vi "getAvailableDevices.vi"(8 "error in (no error)":errorcluster, 11 "IDevice in":refnum<class "IDevice.lvclass">) -> (0 "error out":errorcluster, 2 "availableDeviceInfo out":refnum<class "IDeviceInfo.lvclass">[](array[class]), 3 "IDevice out":refnum<class "IDevice.lvclass">)   [LabVIEW 2022 SP3, in "openDAQ.lvlib" / "IBaseObject.lvlib" / "IPropertyObject.lvlib" / "IComponent.lvlib" / "IFolder.lvlib" / "IDevice.lvlib" / "IDevice.lvclass"]
uses:
  <instrlib>/openDAQ/Public/Classes/IDevice/IDevice.lvclass
  C:/Program Files (x86)/National Instruments/LabVIEW 2022/instr.lib/openDAQ/Public/Classes/IBaseObject/IBaseObject.lvclass
  <instrlib>/openDAQ/Public/Classes/IDeviceInfo/IDeviceInfo.lvclass
  <instrlib>/openDAQ/Public/Classes/daqCoreTypes/IList/IList.lvclass
  <instrlib>/openDAQ/Public/Classes/IBaseObject/IBaseObject.lvclass/IBaseObject.ctl
  <instrlib>/openDAQ/Public/Classes/IBaseObject/Accessor/Read reference.vi
  <instrlib>/openDAQ/Public/Classes/IBaseObject/Accessor/Write reference.vi
  <instrlib>/openDAQ/Public/Classes/daqCoreTypes/IList/Polymorphic/getList/getDeviceInfoList.vi
  <instrlib>/openDAQ/Binaries/Windows/x86/copendaq32.dll
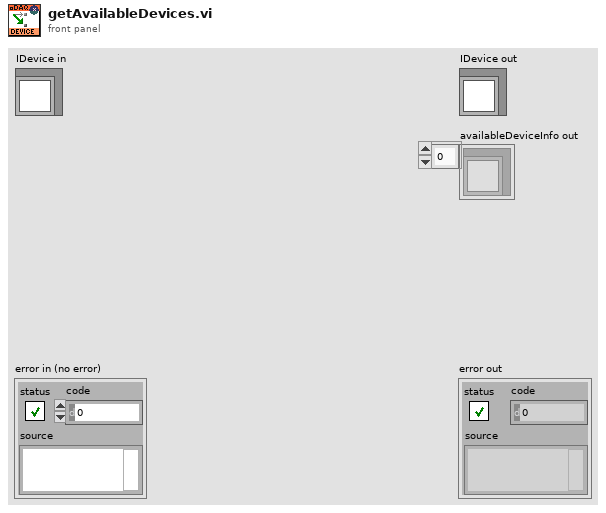
[diagram p1: front panel]
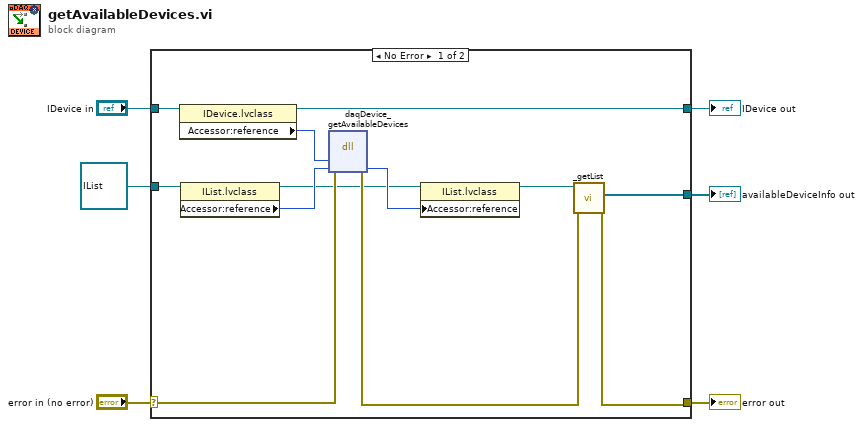
[diagram p0: block diagram]
diagram:
  n1 = case shown="No Error" "error in (no error)" {
    selector: "error in (no error)" -> [w12 w20]
    tunnel: [w8 w20] -> w5
    tunnel: [w17 w19] -> w3
    tunnel: "IDevice in" -> [w18 w19]
    tunnel: refnum<class "IList.lvclass"> refnum ("openDAQ.lvlib:daqCoreTypes.lvlib:IList.lvclass") -> [w15 _]
    tunnel: [w10 _] -> w1
    frame No Error {
      n2 = property class="IDevice.lvclass"(reference=w18) -> (reference out=w17:refnum<class "IDevice.lvclass">, "Accessor:reference"=w16:i64)  [unwired: 1 in, 1 out]
      n3 = property class="IList.lvclass"(reference=w15) -> (reference out=w7:refnum<class "IList.lvclass">, "Accessor:reference"=w14:i64)  [unwired: 1 in, 1 out]
      n4 = dll-call lib="C:/Program Files (x86)/National Instruments/LabVIEW 2022/instr.lib/openDAQ/Binaries/Windows/x86/copendaq*.*" fn="daqDevice_getAvailableDevices"(error in=w12, "instance"=w16, "availableDevices"=w14) -> (error out=w9:errorcluster, "availableDevices"=w13:i64)  [unwired: 4 in, 1 out]
      n5 = property class="IList.lvclass"(reference=w7, "Accessor:reference"=w13) -> (reference out=w11:refnum<class "IList.lvclass">)  [unwired: 1 in, 1 out]
      n6 = call-poly <instrlib>:"_getList.vi"("error in (no error)"=w9, "IList in"=w11) -> ("error out"=w8:errorcluster, "deviceInfos out"=w10:refnum<class "IDeviceInfo.lvclass">[])  [unwired: 8 in]
    }
    frame Error {
    }
  }
  "error out" <- w5
  "IDevice out" <- w3
  "availableDeviceInfo out" <- w1
